vi "Ghost Bus - Tool.vi"() -> ()   [LabVIEW 2019, in "Ghost Bus Tool.lvlib"]
uses:
  Ghost Bus Tool.lvlib
  NationalInstruments.VeriStand.SystemStorage
  SubModules/CAN-Streaming-Support/Source/Addon/Addon Shared/Types/Direction Filter.ctl
  SubModules/CAN-Streaming-Support/Source/Addon/Addon Shared/Types/Type Filter.ctl
  Workspace Shared/Types/Workspace.State.ctl
  Workspace Shared/Types/UI.Refs.ctl
  <vilib>/NI VeriStand/Display Template Support/DisplayTemplateSupport.llb/enum_Display Template Handler Minimal To Workspace.ctl
  Workspace Shared/Types/Workspace.SavedState.ctl
  <vilib>/NI VeriStand/Execution/Workspace/WorkspaceAPI.ctl
  <vilib>/NI VeriStand/Display Template Support/DisplayTemplateSupport.llb/enum_Display Template Handler Minimal To Widget Msg.ctl
  <vilib>/NI VeriStand/Execution/Workspace/SystemStateRegEventRef.ctl
  <vilib>/NI VeriStand/Execution/Workspace/Target State Info.ctl
  <vilib>/NI VeriStand/Execution/Workspace/Target State.ctl
  <vilib>/NI VeriStand/Execution/Workspace/SystemStateEventRef.ctl
  SubModules/CAN-Streaming-Support/Source/UIs/Workspace Shared/Types/Host Stream Queue Refs.ctl
  SubModules/CAN-Streaming-Support/Source/UIs/Workspace Shared/Types/Host Stream Queue Type.ctl
  SubModules/CAN-Streaming-Support/Source/UIs/Workspace Shared/Types/Host Stream Queue Command.ctl
  <vilib>/xnet/xnet.llb/XNET Frame CAN.ctl
  <vilib>/xnet/xnet.llb/XNET Frame Type CAN.ctl
  SubModules/CAN-Streaming-Support/Source/UIs/Workspace Shared/Types/Host Stream Engine Parameters.ctl
  SubModules/CAN-Streaming-Support/Source/Addon/Addon Shared/Types/Filter Parameters.ctl
  <vilib>/Utility/miscctls.llb/LVRowAndColumnUnsignedTypeDef.ctl
  <vilib>/dlg_ctls.llb/Space Constant.vi
  SubModules/CAN-Streaming-Support/Source/UIs/Workspace Shared/SubVIs/Create Host Stream Refs.vi
  SubModules/CAN-Streaming-Support/Source/UIs/Workspace Shared/SubVIs/Read Host Stream.vi
  SubModules/CAN-Streaming-Support/Source/UIs/Workspace Shared/SubVIs/Cleanup Host Stream.vi
  SubModules/CAN-Streaming-Support/Source/UIs/Workspace Shared/SubVIs/Create Bus Log File.vi
  SubModules/CAN-Streaming-Support/Source/UIs/Workspace Shared/SubVIs/Write to Bus Log File.vi
  SubModules/CAN-Streaming-Support/Source/UIs/Workspace Shared/SubVIs/Convert BIN to TXT File.vi
  SubModules/CAN-Streaming-Support/Source/UIs/Workspace Shared/SubVIs/Get Next Bus Engine State.vi
  SubModules/CAN-Streaming-Support/Source/UIs/Workspace Shared/SubVIs/Get Engine Trigger State.vi
  SubModules/CAN-Streaming-Support/Source/UIs/Workspace Shared/SubVIs/Get Next Log Engine State.vi
  SubModules/CAN-Streaming-Support/Source/UIs/Workspace Shared/SubVIs/Process CAN Data.vi
  SubModules/CAN-Streaming-Support/Source/UIs/Workspace Shared/SubVIs/Process CAN State.vi
  SubModules/CAN-Streaming-Support/Source/UIs/Workspace Shared/SubVIs/Convert Frame Array to String Array.vi
  SubModules/CAN-Streaming-Support/Source/UIs/Workspace Shared/SubVIs/Convert Time to UTC String.vi
  <vilib>/Utility/error.llb/Trim Whitespace.vi
  <userlib>/_OpenG.lib/array/array.llb/Sort Array__ogtk.vi
  <userlib>/_OpenG.lib/array/array.llb/Sort 2D Array (String)__ogtk.vi
  <vilib>/Utility/libraryn.llb/Check if File or Folder Exists.vi
  <vilib>/Utility/libraryn.llb/Get File Extension.vi
  Workspace Shared/Ghost Bus Workspace Shared.lvlib
  APIs/Host Automation API/Ghost Bus Host Automation API.lvlib
  <vilib>/NI VeriStand/Execution/Workspace/NI_VS Workspace ExecutionAPI.lvlib
  SubModules/CAN-Streaming-Support/Source/UIs/Workspace Shared/CAN Stream Support Workspace Shared.lvlib
  SubModules/CAN-Streaming-Support/Source/Addon/Addon Shared/CAN Stream Support Shared.lvlib
  NationalInstruments.VeriStand.ClientAPI
panel:
  out "Device":string
  in  "Tab Control":enum32{"Bus Stream", "RAW"}(tab)
  in  "Reset Filter":bool
  in  "Host Filter":bool
  in  "Filter IDs":string caption="Filter IDs (format = x<ID>, comma separated, ID x0 = Bus Error)"
  in  "Clear History":bool
  in  "Type Filter":T1
  out "Table Control":string[][](table)
  in  "Enable Stream":bool
  in  "Pause":bool
  in  "Sort By ID":bool
  out "Stream Connected":bool
  out "Status":string
  in  "Direction Filter":T2
  in  "Log":bool
  in  "Extended?":bool
  in  "Identifier":u32 format="%x"
  in  "Raw Bytes":u8[](array[numeric]) format="%.0x"
  in  "Type":T3(ring)
  out "Error":errorcluster
  in  "Clear Raw":bool
  in  "Send Raw":bool
  in  "NIVS.Gateway IP Address":string
  in  "NIVS.System Definition Root":refnum<k24>
  in  "NIVS.Workspace Event":refnum<event-registration>
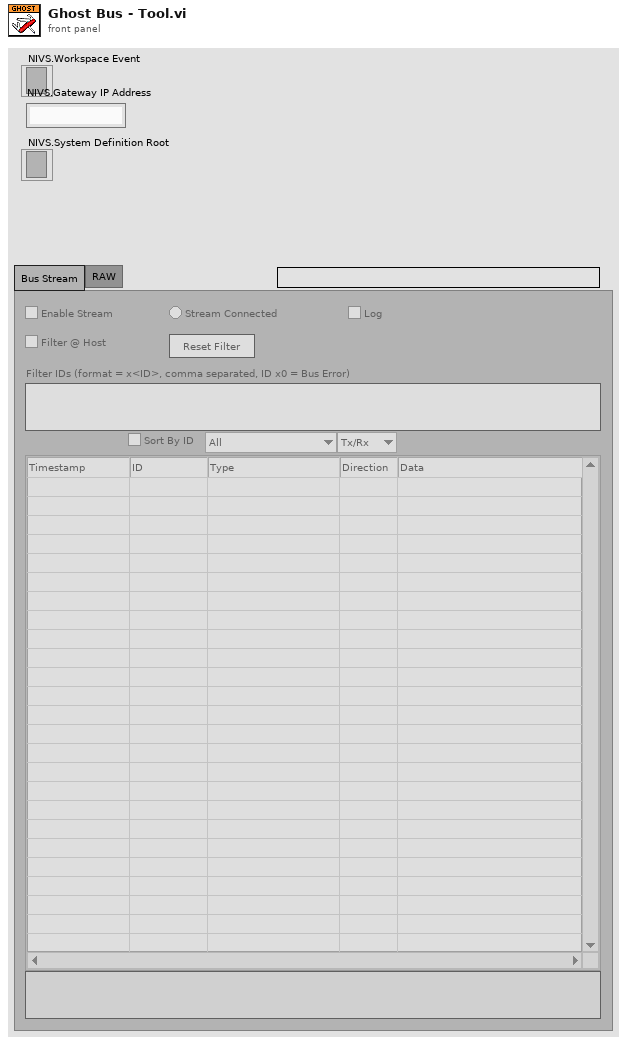
[diagram p1: front panel]
types:
  T1 = typedef "CAN Stream Support Shared.lvlib/Type Filter.ctl" = enum16{"All", "CAN Data", "CAN Remote", "CAN Bus Error", "CAN 2.0 Data", "CAN FD Data", "CAN FD+BRS Data", "J1939 Data", "Delay", "Log Trigger", "Start Trigger"}
  T2 = typedef "CAN Stream Support Shared.lvlib/Direction Filter.ctl" = enum16{"Tx/Rx", "Rx", "Tx"}
  T3 = enum16{"CAN Data", "CAN Remote", "CAN Bus Error", "CAN 2.0 Data", "CAN FD Data", "CAN FD+BRS Data", "J1939 Data", "Delay", "Log Trigger", "Start Trigger"}
  T4 = typedef "Ghost Bus Workspace Shared.lvlib/Workspace.State.ctl" = cluster{"UI.Refs":T5, "CachedData.UserEvent":refnum<user-event>, "CachedData":T6, "Addon.Connected?":bool, "NIVS.SysDef":path, "NIVS.SysDefRoot":refnum<k24>, "NIVS.Workspace":T7, "NIVS.UserEventRefs":cluster{"Event Registration Refnum":refnum<event-registration>, "SystemChangeEventRef":T8, "NIVS.Workspace Event":refnum<event-registration>}, "NIVS.SystemStateRefs":T9, "NIVS.LaunchRef":refnum<user-event>, "Mode.Tool?":bool, "Stream.Qs":T10}
  T5 = typedef "Ghost Bus Workspace Shared.lvlib/UI.Refs.ctl" = cluster{"Device":refnum<vi>, "Pause":refnum<vi>, "Table Control":refnum<vi>, "Sort By ID":refnum<vi>, "Streaming Connected":refnum<vi>, "Enable Stream":refnum<vi>, "CAN State":refnum<vi>, "Direction Filter":refnum<vi>, "Type Filter":refnum<vi>, "Clear History":refnum<vi>, "Filter IDs":refnum<vi>, "Filter Location":refnum<vi>, "Reset Filter":refnum<vi>, "Log":refnum<vi>, "Type":refnum<vi>, "Extended?":refnum<vi>, "Identifier":refnum<vi>, "Raw Bytes":refnum<vi>, "Send Raw":refnum<vi>, "Clear Raw":refnum<vi>, "Raw Error":refnum<vi>}
  T6 = typedef "Ghost Bus Workspace Shared.lvlib/Workspace.SavedState.ctl" = cluster{"CD Path":string, "CD IP":string}
  T7 = typedef "NI_VS Workspace ExecutionAPI.lvlib/WorkspaceAPI.ctl" = refnum<k24>
  T8 = typedef "NI_VS Workspace ExecutionAPI.lvlib/SystemStateRegEventRef.ctl" = refnum<event-registration>
  T9 = typedef "NI_VS Workspace ExecutionAPI.lvlib/SystemStateEventRef.ctl" = cluster{"CustDatRef":refnum<user-event>, "EvtRef":refnum<k27>, "Target State User Event":refnum<user-event>}
  T10 = typedef "CAN Stream Support Workspace Shared.lvlib/Host Stream Queue Refs.ctl" = cluster{"Cmd Q":refnum<queue>, "XNET Frames":refnum<queue>}
  T11 = typedef "enum_Display Template Handler Minimal To Workspace.ctl" = cluster{"Operation":enum16{"SetCustomData", "DeleteItem"}, "Data":variant}
  T12 = typedef "XNET Frame CAN.ctl" = cluster{"timestamp":timestamp, "payload":u8[], "identifier":u32, "type":T13, "extended?":bool, "echo?":bool}
  T13 = typedef "XNET Frame Type CAN.ctl" = u8
  T14 = typedef "CAN Stream Support Shared.lvlib/Filter Parameters.ctl" = cluster{"ID Filters":u32[], "Direction Filter":T2, "Type Filter":T1}
  T15 = typedef "LVRowAndColumnUnsignedTypeDef.ctl" = cluster{"Row":u32, "Column":u32}
  T16 = cluster{"Event Registration Refnum":refnum<event-registration>, "SystemChangeEventRef":T8, "NIVS.Workspace Event":refnum<event-registration>}
  T17 = typedef "enum_Display Template Handler Minimal To Widget Msg.ctl" = enum16{"Stop", "LaunchConfigDialog"}
  T18 = enum8{"Enabled", "Disabled", "Disabled and Grayed Out"}
  T19 = typedef "Ghost Bus Host Automation API.lvlib/API Variables.ctl" = cluster{"TCP Comm":T20}
  T20 = typedef "NI STM.lvlib/TCP Connection Info.ctl" = cluster{"connection ID":refnum<k5>, "meta data":T21[]}
  T21 = typedef "NI STM.lvlib/MetaDataElement.ctl" = string
  T22 = typedef "CAN Stream Support Workspace Shared.lvlib/Host Stream Engine Parameters.ctl" = cluster{"Host Filter":bool, "Filter Parameters":T14, "Sort By ID":bool, "Pause":bool, "Clear History":bool, "Log":bool}
  T23 = typedef "CAN Stream Support Workspace Shared.lvlib/Host Stream Data.ctl" = cluster{"Connected":bool, "Bus Data Update":bool, "Bus Data":string[][], "Bus Status":string, "Bus Warning":bool, "Log Status":string}
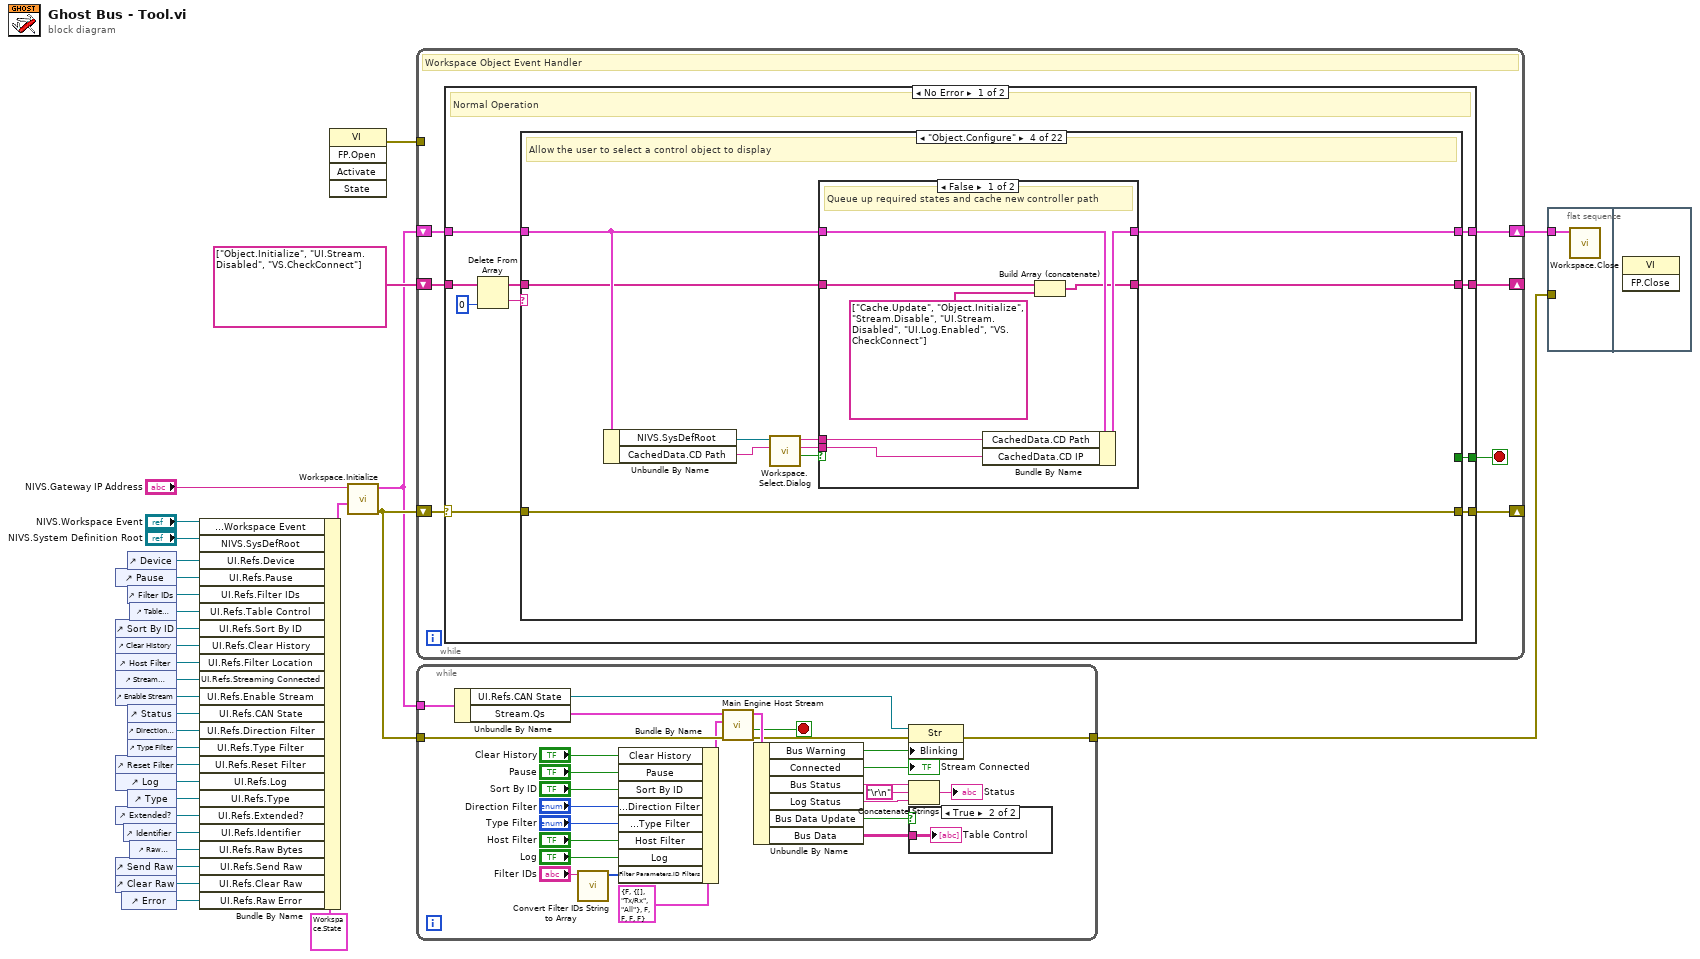
[diagram p0: block diagram]
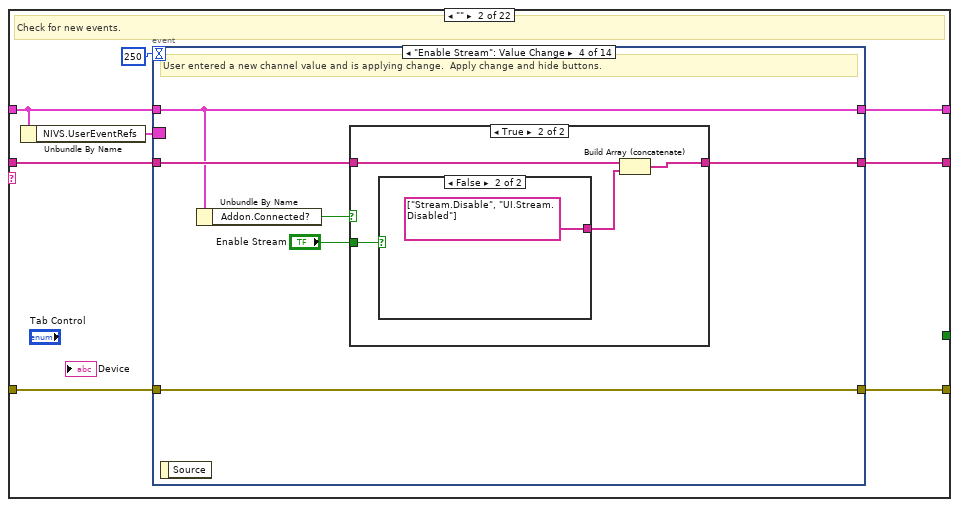
[diagram p4: hidden frame]
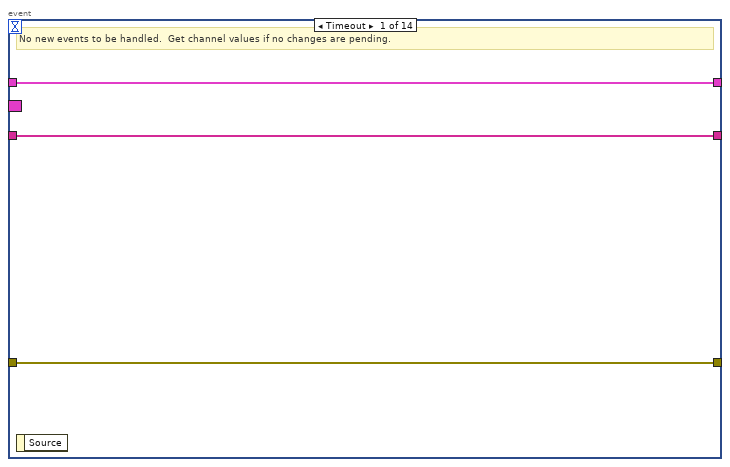
[diagram p5: hidden frame]
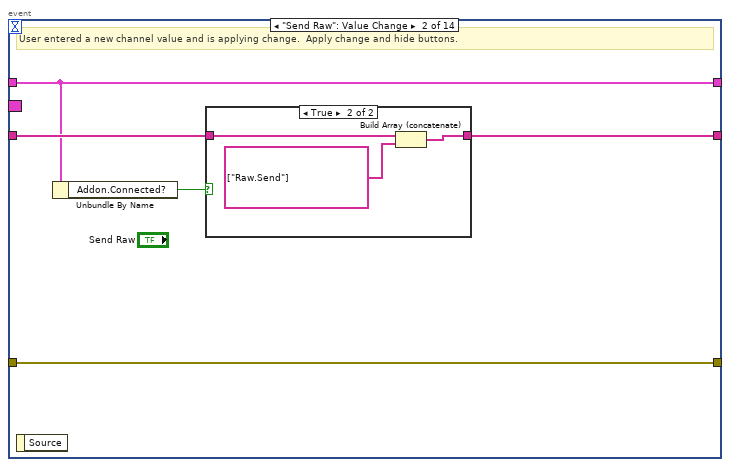
[diagram p6: hidden frame]
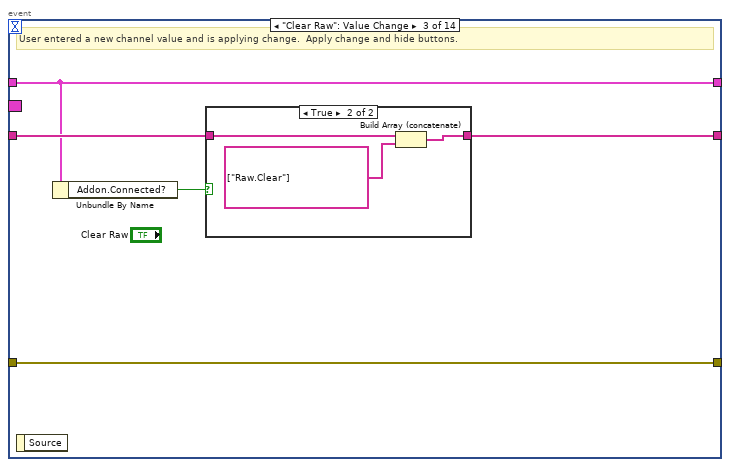
[diagram p8: hidden frame]
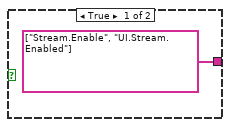
[diagram p11: hidden frame]
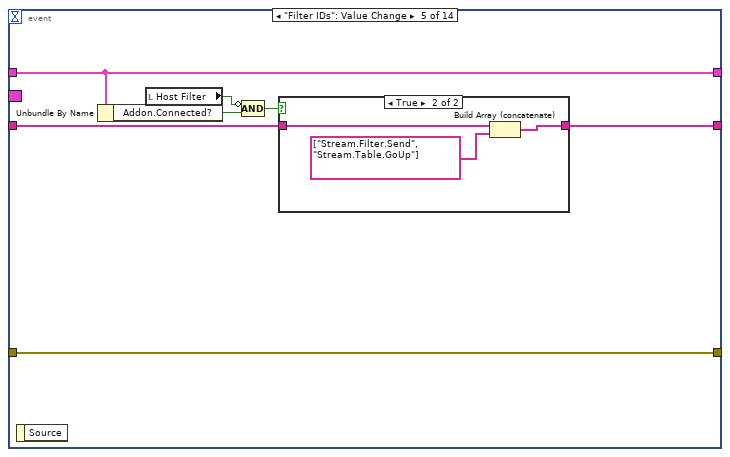
[diagram p12: hidden frame]
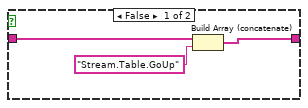
[diagram p13: hidden frame]
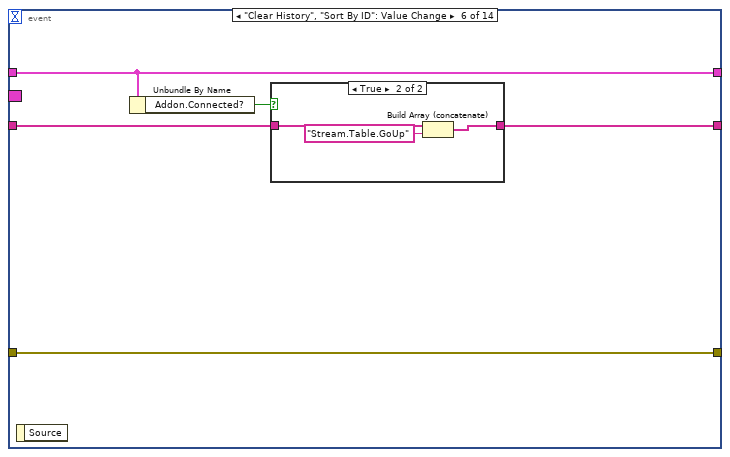
[diagram p14: hidden frame]
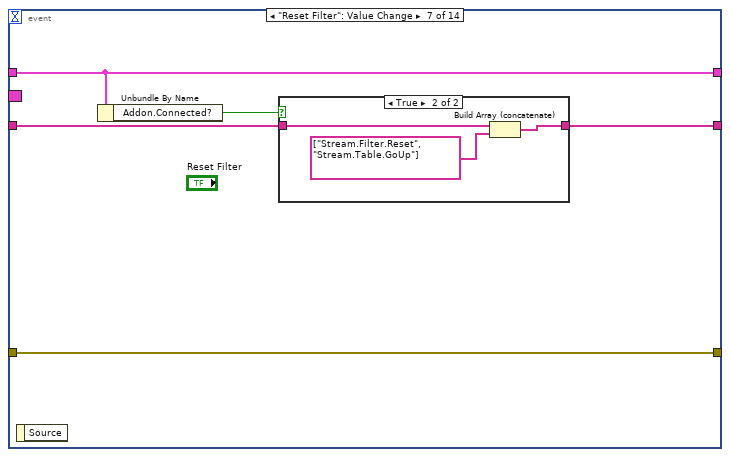
[diagram p16: hidden frame]
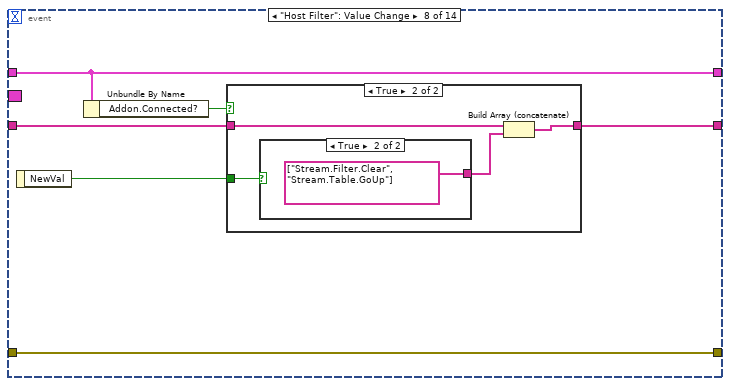
[diagram p18: hidden frame]
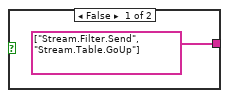
[diagram p20: hidden frame]
diagram:
  n1 = control-ref of="Pause"() -> (w23:refnum<vi>)
  n2 = control-ref of="Sort By ID"() -> (w21:refnum<vi>)
  n3 = control-ref of="Clear History"() -> (w11:refnum<vi>)
  n4 = control-ref of="Host Filter"() -> (w10:refnum<vi>)
  n5 = control-ref of="Stream Connected"() -> (w20:refnum<vi>)
  n6 = control-ref of="Enable Stream"() -> (w19:refnum<vi>)
  n7 = control-ref of="Reset Filter"() -> (w9:refnum<vi>)
  n8 = control-ref of="Log"() -> (w8:refnum<vi>)
  n9 = control-ref of="Extended?"() -> (w4:refnum<vi>)
  n10 = control-ref of="Send Raw"() -> (w1:refnum<vi>)
  n11 = control-ref of="Clear Raw"() -> (w2:refnum<vi>)
  n12 = control-ref of="Error"() -> (w3:refnum<vi>)
  n13 = control-ref of="Identifier"() -> (w5:refnum<vi>)
  n14 = control-ref of="Device"() -> (w24:refnum<vi>)
  n15 = control-ref of="Filter IDs"() -> (w12:refnum<vi>)
  n16 = control-ref of="Status"() -> (w18:refnum<vi>)
  n17 = control-ref of="Direction Filter"() -> (w14:refnum<vi>)
  n18 = control-ref of="Type Filter"() -> (w13:refnum<vi>)
  n19 = control-ref of="Type"() -> (w7:refnum<vi>)
  n20 = control-ref of="Table Control"() -> (w22:refnum<vi>)
  n21 = control-ref of="Raw Bytes"() -> (w6:refnum<vi>)
  n22 = Bundle By Name(cluster=T4 {"UI.Refs"={"Device"=refnum, "Pause"=refnum, "Table Control"=refnum, "Sort By ID"=refnum, "Streaming Connected"=refnum, "Enable Stream"=refnum, "CAN State"=refnum, "Direction Filter"=refnum, "Type Filter"=refnum, "Clear History"=refnum, "Filter IDs"=refnum, "Filter Location"=refnum, "Reset Filter"=refnum, "Log"=refnum, "Type"=refnum, "Extended?"=refnum, "Identifier"=refnum, "Raw Bytes"=refnum, "Send Raw"=refnum, "Clear Raw"=refnum, "Raw Error"=refnum}, "CachedData.UserEvent"=refnum, "CachedData"={"CD Path"="", "CD IP"=""}, "Addon.Connected?"=FALSE, "NIVS.SysDef"=path "", "NIVS.SysDefRoot"=refnum, "NIVS.Workspace"=refnum, "NIVS.UserEventRefs"={"Event Registration Refnum"=refnum, "SystemChangeEventRef"=refnum, "NIVS.Workspace Event"=refnum}, "NIVS.SystemStateRefs"={"CustDatRef"=refnum, "EvtRef"=refnum, "Target State User Event"=refnum}, "NIVS.LaunchRef"=refnum, "Mode.Tool?"=FALSE, "Stream.Qs"={"Cmd Q"=refnum, "XNET Frames"=refnum}}, "NIVS.UserEventRefs.NIVS.Workspace Event"="NIVS.Workspace Event", "NIVS.SysDefRoot"="NIVS.System Definition Root", "UI.Refs.Device"=w24, "UI.Refs.Pause"=w23, "UI.Refs.Filter IDs"=w12, "UI.Refs.Table Control"=w22, "UI.Refs.Sort By ID"=w21, "UI.Refs.Clear History"=w11, "UI.Refs.Filter Location"=w10, "UI.Refs.Streaming Connected"=w20, "UI.Refs.Enable Stream"=w19, "UI.Refs.CAN State"=w18, "UI.Refs.Direction Filter"=w14, "UI.Refs.Type Filter"=w13, "UI.Refs.Reset Filter"=w9, "UI.Refs.Log"=w8, "UI.Refs.Type"=w7, "UI.Refs.Extended?"=w4, "UI.Refs.Identifier"=w5, "UI.Refs.Raw Bytes"=w6, "UI.Refs.Send Raw"=w1, "UI.Refs.Clear Raw"=w2, "UI.Refs.Raw Error"=w3) -> (w30:T4)
  n23 = invoke class="VI" method="FP.Open"() -> (error out=w28:errorcluster)  [unwired: 5 in, 4 out]
  n24 = call "Workspace.Initialize.vi"("State Variables in"=w30, "NIVS.Gateway IP Address"="NIVS.Gateway IP Address") -> ("error out"=w17:errorcluster, "State Variables out"=w16:T4)  [unwired: 8 in]
  n25 = while {
    shift-right: [w37] -> _
    shift-left: string[] ["Object.Initialize", "UI.Stream.Disabled", "VS.CheckConnect"] -> [w38]
    shift-right: [w35] -> w27
    shift-left: w16 -> [w34]
    shift-right: [w36] -> _
    shift-left: w17 -> [w33]
    tunnel: w28 -> [_]
    stop <- w39 stop-if-true
    # "Workspace Object Event Handler"
    n26 = case shown="No Error" w33 {
      selector: w33 -> [w40 w431]
      tunnel: [w49 _] -> w39
      tunnel: w38 -> [w47 w438]
      tunnel: [w44 w438] -> w37
      tunnel: [w43 w429] -> w36
      tunnel: [w42 w437] -> w35
      tunnel: w34 -> [w41 w437]
      frame No Error {
        # "Normal Operation"
        n27 = Delete From Array(array=w47, index=0) -> (deleted portion=w46:string, array with subset deleted=w45:string[])  [unwired: 1 in]
        n28 = case shown="\"Object.Configure\"" w46 {
          tunnel: [_ _ _ _ _ _ _ TRUE _ _ _ _ _ _ _ _ _ _ _ _ _ _] -> w49
          tunnel: [w52 w59 w210 w215 w236 w242 w248 w269 w276 w280 w294 w307 w320 w341 w345 w354 w372 w384 w401 w417 w423 w428] -> w44
          tunnel: w40 -> [w51 w57 w205 w221 w231 w240 w253 w266 w275 w278 w291 w305 w317 w340 w344 w353 w365 w377 w394 w408 w418 w424]
          tunnel: w45 -> [w52 w58 w210 w214 w236 w242 w247 w269 w276 w280 w294 w307 w320 w341 w345 w354 w372 w384 w401 w417 w423 w428]
          tunnel: w41 -> [w50 w53 w209 w219 w232 w239 w245 w265 w272 w277 w293 w306 w319 w337 w343 w351 w368 w380 w397 w411 w422 w427]
          tunnel: [w51 w56 w207 w221 w234 w237 w252 w267 w275 w279 w282 w304 w309 w340 w344 w352 w365 w377 w394 w408 w419 w425] -> w43
          tunnel: [w50 w55 w209 w218 w233 w238 w246 w265 w272 w277 w293 w306 w319 w337 w343 w351 w368 w380 w397 w411 w422 w427] -> w42
          frame Default {
            # "Do nothing."
          }
          frame "" {
            # "Check for new events."
            n29 = Unbundle By Name(w53) -> ("NIVS.UserEventRefs"=w54:T16)
            n30 = event shown="[3] \"Enable Stream\": Value Change" {
              selector: w54 -> [_ _ _ _ _ _ _ _ _ _ _ _ _ _]
              dyn-events: _ -> [_ _ _ _ _ _ _ _ _ _ _ _ _ _]
              timeout: 250 -> [_ _ _ _ _ _ _ _ _ _ _ _ _ _]
              tunnel: [w61 w66 w75 w85 w100 w111 w120 w130 w143 w153 w166 w182 w194 w201] -> w59
              tunnel: w58 -> [w61 w67 w76 w86 w99 w110 w119 w129 w142 w155 w165 w181 w195 w202]
              tunnel: w57 -> [w63 w68 w77 w87 w101 w112 w121 w131 w144 w152 w173 w180 w198 w204]
              tunnel: [w63 w68 w77 w87 w101 w112 w121 w131 w144 w152 w173 w180 w198 w204] -> w56
              tunnel: [w62 w65 w74 w84 w98 w109 w118 w128 w141 w157 w172 w178 w197 w203] -> w55
              tunnel: w53 -> [w62 w65 w74 w84 w98 w109 w118 w128 w141 w157 w172 w179 w197 w203]
              event Timeout {
                # "No new events to be handled.  Get channel values if no changes are pending."
                n31 = event-data() -> ()  [unwired: 2 out]
              }
              event "Send Raw": Value Change {
                # "User entered a new channel value and is applying change.  Apply change and hide buttons."
                n32 = event-data() -> ()  [unwired: 2 out]
                n33 = Unbundle By Name(w65) -> ("Addon.Connected?"=w64:bool)
                n34 = case shown="True" w64 {
                  tunnel: w67 -> [w69 w71]
                  tunnel: [w69 w70] -> w66
                  frame False {
                  }
                  frame True {
                    n35 = Build Array (concatenate)(w71, string[] ["Raw.Send"]) -> (w70:string[])
                  }
                }
              }
              event "Clear Raw": Value Change {
                # "User entered a new channel value and is applying change.  Apply change and hide buttons."
                n36 = event-data() -> ()  [unwired: 2 out]
                n37 = Unbundle By Name(w74) -> ("Addon.Connected?"=w73:bool)
                n38 = case shown="True" w73 {
                  tunnel: w76 -> [w78 w80]
                  tunnel: [w78 w79] -> w75
                  frame False {
                  }
                  frame True {
                    n39 = Build Array (concatenate)(w80, string[] ["Raw.Clear"]) -> (w79:string[])
                  }
                }
              }
              event "Enable Stream": Value Change {
                # "User entered a new channel value and is applying change.  Apply change and hide buttons."
                n40 = event-data() -> ()  [unwired: 2 out]
                n41 = Unbundle By Name(w84) -> ("Addon.Connected?"=w83:bool)
                n42 = case shown="True" w83 {
                  tunnel: w86 -> [w88 w91]
                  tunnel: [w88 w90] -> w85
                  tunnel: "Enable Stream" -> [_ w89]
                  frame False {
                  }
                  frame True {
                    n43 = case shown="False" w89 {
                      tunnel: [string[] ["Stream.Enable", "UI.Stream.Enabled"] string[] ["Stream.Disable", "UI.Stream.Disabled"]] -> w92
                      frame True {
                      }
                      frame False {
                      }
                    }
                    n44 = Build Array (concatenate)(w91, w92) -> (w90:string[])
                  }
                }
              }
              event "Filter IDs": Value Change {
                n45 = event-data() -> ()  [unwired: 2 out]
                n46 = Unbundle By Name(w98) -> ("Addon.Connected?"=w96:bool)
                n47 = local read "Host Filter"() -> (w97:bool)
                n48 = Compound Arithmetic op=AND(invert w97, w96) -> (w95:bool)
                n49 = case shown="True" w95 {
                  tunnel: w99 -> [w102 w106]
                  tunnel: [w103 w105] -> w100
                  frame False {
                    n50 = Build Array (concatenate)(w102, "Stream.Table.GoUp") -> (w103:string[])
                  }
                  frame True {
                    n51 = Build Array (concatenate)(w106, string[] ["Stream.Filter.Send", "Stream.Table.GoUp"]) -> (w105:string[])
                  }
                }
              }
              event "Clear History", "Sort By ID": Value Change {
                n52 = event-data() -> ()  [unwired: 2 out]
                n53 = Unbundle By Name(w109) -> ("Addon.Connected?"=w108:bool)
                n54 = case shown="True" w108 {
                  tunnel: [w113 w116] -> w111
                  tunnel: w110 -> [w113 w115]
                  frame False {
                  }
                  frame True {
                    n55 = Build Array (concatenate)(w115, "Stream.Table.GoUp") -> (w116:string[])
                  }
                }
              }
              event "Reset Filter": Value Change {
                n56 = event-data() -> ()  [unwired: 2 out]
                n57 = Unbundle By Name(w118) -> ("Addon.Connected?"=w117:bool)
                n58 = case shown="True" w117 {
                  tunnel: w119 -> [w122 w124]
                  tunnel: [w122 w123] -> w120
                  frame False {
                  }
                  frame True {
                    n59 = Build Array (concatenate)(w124, string[] ["Stream.Filter.Reset", "Stream.Table.GoUp"]) -> (w123:string[])
                  }
                }
              }
              event "Host Filter": Value Change {
                n60 = event-data() -> ("NewVal"=w126:bool)  [unwired: 1 out]
                n61 = Unbundle By Name(w128) -> ("Addon.Connected?"=w127:bool)
                n62 = case shown="True" w127 {
                  tunnel: w129 -> [w132 w135]
                  tunnel: [w132 w134] -> w130
                  tunnel: w126 -> [_ w133]
                  frame False {
                  }
                  frame True {
                    n63 = case shown="True" w133 {
                      tunnel: [string[] ["Stream.Filter.Send", "Stream.Table.GoUp"] string[] ["Stream.Filter.Clear", "Stream.Table.GoUp"]] -> w136
                      frame False {
                      }
                      frame True {
                      }
                    }
                    n64 = Build Array (concatenate)(w135, w136) -> (w134:string[])
                  }
                }
              }
              event "Log": Value Change {
                n65 = event-data() -> ("NewVal"=w139:bool)  [unwired: 1 out]
                n66 = Unbundle By Name(w141) -> ("Addon.Connected?"=w140:bool)
                n67 = case shown="True" w140 {
                  tunnel: w142 -> [w145 w148]
                  tunnel: [w145 w147] -> w143
                  tunnel: w139 -> [_ w146]
                  frame False {
                  }
                  frame True {
                    n68 = case shown="False" w146 {
                      tunnel: [string[] ["UI.Log.Disabled"] string[] ["UI.Log.Enabled"]] -> w149
                      frame False {
                      }
                      frame True {
                      }
                    }
                    n69 = Build Array (concatenate)(w148, w149) -> (w147:string[])
                  }
                }
              }
              event User Event {
                # "System state has changed. Handle accordingly."
                n70 = event-data() -> ("SystemStateChange"=w156:string)  [unwired: 1 out]
                n71 = Unbundle By Name(w157) -> ("Mode.Tool?"=w158:bool)
                n72 = case shown="True" w158 {
                  tunnel: ["VS.CheckConnect" w161] -> w154
                  tunnel: w156 -> [_ w160]
                  frame False {
                  }
                  frame True {
                    n73 = case shown="\"Stop Configuration\"" w160 {
                      tunnel: ["Object.Exit" "VS.CheckConnect"] -> w161
                      frame "Stop Configuration" {
                      }
                      frame Default {
                      }
                    }
                  }
                }
                n74 = Build Array (concatenate)(w155, w154) -> (w153:string[])
              }
              event User Event {
                n75 = event-data() -> ("Workspace Event"=w167:string)  [unwired: 1 out]
                n76 = Equal?(x=w167, y="Shut Down") -> (x = y?=w168:bool)
                n77 = Equal?(x=w167, y="Disconnect") -> (x = y?=w169:bool)
                n78 = Compound Arithmetic op=OR(w168, w169) -> (w164:bool)
                n79 = case shown="True" w164 {
                  tunnel: [w174 w176] -> w166
                  tunnel: w165 -> [w174 w175]
                  frame False {
                  }
                  frame True {
                    n80 = Build Array (concatenate)(w175, "Object.Exit") -> (w176:string[])
                  }
                }
              }
              event User Event {
                # "Widget event has occurred.  Handle accordingly."
                n81 = event-data() -> ("ToWidgetMessage"=w183:T17)  [unwired: 1 out]
                n82 = case shown="\"Stop\"" w183 {
                  tunnel: [w185 w188 w192] -> w182
                  tunnel: w181 -> [w185 w189 w193]
                  tunnel: w179 -> [w184 w186 w190]
                  tunnel: [w184 w186 w190] -> w178
                  frame Default {
                    # "Do nothing."
                  }
                  frame "Stop" {
                    # "User exiting workspace or deleting object"
                    n83 = Build Array (concatenate)(w189, "Object.Exit") -> (w188:string[])
                  }
                  frame "LaunchConfigDialog" {
                    # "User wants to configure object"
                    n84 = Build Array (concatenate)(w193, "Object.Configure") -> (w192:string[])
                  }
                }
              }
              event Menu Selection (User) {
                n85 = event-data() -> ("ItemTag"=w196:string)  [unwired: 1 out]
                n86 = Build Array (concatenate)(w195, w196) -> (w194:string[])
              }
              event Panel Close? {
                n87 = event-data() -> ()  [unwired: 5 out]
                n88 = Build Array (concatenate)(w202, "Object.Exit") -> (w201:string[])
                n89 = event-data("Discard?"=TRUE) -> ()  [unwired: 1 in, 1 out]
              }
            }
          }
          frame "Object.Initialize" {
            # "Initialize the workspace Object state variables and UI"
            n90 = local write "Tab Control"(0) -> ()
            n91 = Unbundle By Name(w209) -> ("UI.Refs.Filter Location"=w206:refnum<vi>)
            n92 = property class="Bool (strict)"(reference=w206, error in=w205, "Value"=FALSE) -> (error out=w207:errorcluster)  [unwired: 1 out]
          }
          frame "Object.Configure" {
            # "Allow the user to select a control object to display"
            n93 = Unbundle By Name(w219) -> ("NIVS.SysDefRoot"=w213:refnum<k24>, "CachedData.CD Path"=w220:string)
            n94 = call "Workspace.Select.Dialog.vi"("CD Path"=w220, "NIVS.System Definition Root"=w213) -> ("Cancelled?"=w217:bool, "IP Address"=w212:string, "Custom Device Path Out"=w216:string)  [unwired: 7 in]
            n95 = case shown="False" w217 {
              tunnel: w219 -> [w228 w229]
              tunnel: [w227 w229] -> w218
              tunnel: w216 -> [w226 _]
              tunnel: [w224 w230] -> w215
              tunnel: w214 -> [w225 w230]
              tunnel: w212 -> [w222 _]
              frame False {
                # "Queue up required states and cache new controller path"
                n96 = Bundle By Name(cluster=w228, "CachedData.CD Path"=w226, "CachedData.CD IP"=w222) -> (w227:T4)
                n97 = Build Array (concatenate)(w225, string[] ["Cache.Update", "Object.Initialize", "Stream.Disable", "UI.Stream.Disabled", "UI.Log.Enabled", "VS.CheckConnect"]) -> (w224:string[])
              }
              frame True {
                # "User canceled"
              }
            }
          }
          frame "Object.Connected" {
            # "System state is Connected. Get path to required channels and start UDP acquisition if channels found."
            n98 = call "Workspace.UI.DisableState.Set.vi"("Enable?"=TRUE, "error in (no error)"=w231, "State Variables in"=w232) -> ("error out"=w234:errorcluster, "State Variables out"=w233:T4)  [unwired: 7 in]
          }
          frame "Object.Disconnected" {
            n99 = call "Workspace.UI.DisableState.Set.vi"("Enable?"=FALSE, "error in (no error)"=w240, "State Variables in"=w239) -> ("error out"=w237:errorcluster, "State Variables out"=w238:T4)  [unwired: 7 in]
          }
          frame "VS.CheckConnect" {
            n100 = Unbundle By Name(w245) -> ("UI.Refs.Device"=w244:refnum<vi>, "NIVS.Workspace"=w256:T7, "NIVS.SysDefRoot"=w255:refnum<k24>, "CachedData.CD Path"=w254:string)
            n101 = Current VI's Menubar() -> (w257:refnum<k9>)
            n102 = call "UI.Connection.State.Get.vi"("Menu Ref"=w257, "Name Ref"=w244, "error in (no error)"=w253, "Addon Path in"=w254, "NIVS.System Definition Root in"=w255, "NIVS.Workspace Ref in"=w256) -> ("error out"=w252:errorcluster, "Addon Connected?"=w249:bool, "NIVS.System Definition Root out"=w250:refnum<k24>, "NIVS.Workspace Ref out"=w251:T7, "System Definition File"=w243:path)  [unwired: 1 in]
            n103 = case shown="True" w249 {
              tunnel: [w260 w263] -> w248
              tunnel: w247 -> [w259 w262]
              frame True {
                # "Addon connected"
                n104 = Build Array (concatenate)(w259, string[] ["Object.Connected", "Stream.Filter.Read"]) -> (w260:string[])
              }
              frame False {
                # "Addon not connected"
                n105 = Build Array (concatenate)(w262, string[] ["Object.Disconnected", "UI.Stream.Disabled", "Stream.Disable"]) -> (w263:string[])
              }
            }
            n106 = Bundle By Name(cluster=w245, "NIVS.SysDef"=w243, "NIVS.Workspace"=w251, "NIVS.SysDefRoot"=w250, "Addon.Connected?"=w249) -> (w246:T4)
          }
          frame "Object.Exit" {
            # "Stop current loop.  Queue Stop Acq and Exit to UDP loop."
            n107 = Unbundle By Name(w265) -> ("Stream.Qs"=w264:T10)
            n108 = call "Send Host Stream Command Exit.vi"("error in (no error)"=w266, "Q Refs"=w264) -> ("error out"=w267:errorcluster)  [unwired: 9 in]
          }
          frame "Cache.Update" {
            # "Cache any data needing to be permenantly stored with the workspace object."
            n109 = Unbundle By Name(w272) -> ("CachedData.UserEvent"=w270:refnum<user-event>, "CachedData"=w271:T6)
            n110 = Bundle By Name(cluster=T11 {"Operation"=enum."SetCustomData", "Data"=variant} ("event data"), "Data"=w271) -> (w273:T11)
            n111 = Generate User Event(user event=w270, event data cluster=w273) -> ()  [unwired: 2 in, 2 out]
          }
          frame "UI.Stream.Enabled" {
            n112 = call "UI.Stream.Enable.vi"("error in (no error)"=w278, "State Variables in"=w277) -> ("error out"=w279:errorcluster)  [unwired: 9 in]
          }
          frame "UI.Log.Enabled" {
            w281 = T18."Disabled and Grayed Out" ("Disabled")
            n113 = Unbundle By Name(w293) -> ("UI.Refs.Type Filter"=w286:refnum<vi>, "UI.Refs.Filter IDs"=w285:refnum<vi>, "UI.Refs.Direction Filter"=w284:refnum<vi>, "UI.Refs.Reset Filter"=w289:refnum<vi>, "UI.Refs.Filter Location"=w292:refnum<vi>)
            n114 = property class="Bool (strict)"(reference=w292, error in=w291, "DisabledEnum"=w281) -> (error out=w290:errorcluster, "Value"=w288:bool)  [unwired: 1 out]
            n115 = Build Array(w286, w285, w284) -> (w283:refnum<vi>[])
            n116 = property class="Bool"(reference=w289, error in=w290, "DisabledEnum"=w281) -> (error out=w287:errorcluster)  [unwired: 1 out]
            n117 = case shown="False" w288 {
              tunnel: w287 -> [w297 w303]
              tunnel: w283 -> [w298 _]
              tunnel: [w296 w303] -> w282
              tunnel: w281 -> [w295 _]
              frame False {
                n118 = for {
                  tunnel: w298 -> [w302] mode=indexing
                  shift-right: [w300] -> w296
                  shift-left: w297 -> [w301]
                  tunnel: w295 -> [w299]
                  n119 = property class="Ctl"(reference=w302, error in=w301, "DisabledEnum"=w299) -> (error out=w300:errorcluster)  [unwired: 1 out]
                }
              }
              frame True {
              }
            }
          }
          frame "UI.Stream.Disabled" {
            n120 = call "UI.Stream.Disable.vi"("error in (no error)"=w305, "State Variables in"=w306) -> ("error out"=w304:errorcluster)  [unwired: 9 in]
          }
          frame "UI.Log.Disabled" {
            w308 = T18."Enabled" ("Disabled")
            n121 = Unbundle By Name(w319) -> ("UI.Refs.Type Filter"=w313:refnum<vi>, "UI.Refs.Filter IDs"=w312:refnum<vi>, "UI.Refs.Direction Filter"=w311:refnum<vi>, "UI.Refs.Reset Filter"=w315:refnum<vi>, "UI.Refs.Filter Location"=w318:refnum<vi>)
            n122 = property class="Bool (strict)"(reference=w318, error in=w317, "DisabledEnum"=w308) -> (error out=w316:errorcluster)  [unwired: 1 out]
            n123 = Build Array(w313, w312, w311) -> (w310:refnum<vi>[])
            n124 = property class="Bool"(reference=w315, error in=w316, "DisabledEnum"=w308) -> (error out=w314:errorcluster)  [unwired: 1 out]
            n125 = for {
              tunnel: w310 -> [w324] mode=indexing
              shift-right: [w322] -> w309
              shift-left: w314 -> [w323]
              tunnel: w308 -> [w321]
              n126 = property class="Ctl"(reference=w324, error in=w323, "DisabledEnum"=w321) -> (error out=w322:errorcluster)  [unwired: 1 out]
            }
          }
          frame "Raw.Send" {
            # "Reset slow speed channel displayed values."
            n127 = Unbundle By Name(w337) -> ("CachedData.CD IP"=w335:string, "CachedData.CD Path"=w333:string)
            n128 = call "UI.Addon.Path.Parse.vi"("Cached Addon Path"=w333) -> ("Addon Name"=w332:string)  [unwired: 6 in, 4 out]
            n129 = call "Connect.vi"("Addon Name"=w332, "Address"=w335) -> ("error out"=w336:errorcluster, "Ref"=w338:T19)  [unwired: 8 in]
            n130 = Bundle By Name(cluster=T12 {"timestamp"=timestamp(0 s since 1904-01-01), "payload"=[], "identifier"=0, "type"=0, "extended?"=FALSE, "echo?"=FALSE} ("Frame"), "extended?"="Extended?", "type"="Type", "identifier"="Identifier", "payload"="Raw Bytes") -> (w330:T12)
            n131 = call "PassThru.vi"("error in (no error)"=w336, "timeout ms (1000)"=2500, "Frame"=w330, "Ref in"=w338) -> ("error out"=w331:errorcluster, "Ref out"=w339:T19)  [unwired: 6 in]
            "Error" <- w331
            n132 = call "Disconnect.vi"("error in (no error)"=w331, "Ref"=w339) -> ()  [unwired: 9 in, 1 out]
          }
          frame "Raw.Clear" {
            n133 = local write "Raw Bytes"(u8[] [] ("Cmd")) -> ()
          }
          frame "Stream.Enable" {
            n134 = Unbundle By Name(w351) -> ("Stream.Qs"=w348:T10, "CachedData.CD IP"=w349:string, "CachedData.CD Path"=w355:string, "NIVS.SysDef"=w347:path)
            n135 = Strip Path(path=w347) -> (stripped path=w346:path)  [unwired: 1 out]
            n136 = call "UI.Addon.Path.Parse.vi"("Cached Addon Path"=w355) -> ("Addon Name"=w350:string)  [unwired: 6 in, 4 out]
            n137 = call "Send Host Stream Command Start.vi"("Project Folder"=w346, "error in (no error)"=w353, "Addon"=w350, "Target IP Address"=w349, "Q Refs"=w348) -> ("error out"=w352:errorcluster)  [unwired: 6 in]
          }
          frame "Stream.Filter.Send" {
            n138 = Unbundle By Name(w368) -> ("CachedData.CD IP"=w366:string, "CachedData.CD Path"=w369:string)
            n139 = local read "Direction Filter"() -> (w357:T2)
            n140 = local read "Type Filter"() -> (w358:T1)
            n141 = local read "Filter IDs"() -> (w359:string)
            n142 = call "Convert Filter IDs String to Array.vi"("Filter IDs"=w359) -> ("Filter IDs"=w356:u32[])  [unwired: 10 in]
            n143 = call "UI.Addon.Path.Parse.vi"("Cached Addon Path"=w369) -> ("Addon Name"=w367:string)  [unwired: 6 in, 4 out]
            n144 = Bundle By Name(cluster=T14 {"ID Filters"=[], "Direction Filter"=enum."Tx/Rx", "Type Filter"=enum."All"} ("IDs"), "Direction Filter"=w357, "Type Filter"=w358, "ID Filters"=w356) -> (w360:T14)
            n145 = call "Connect.vi"("Addon Name"=w367, "Address"=w366) -> ("error out"=w363:errorcluster, "Ref"=w362:T19)  [unwired: 8 in]
            n146 = call "SetStreamingFilter.vi"("error in (no error)"=w363, "IDs"=w360, "Ref in"=w362) -> ("error out"=w371:errorcluster, "Ref out"=w370:T19)  [unwired: 7 in]
            n147 = call "Disconnect.vi"("error in (no error)"=w371, "Ref"=w370) -> ("error out"=w364:errorcluster)  [unwired: 9 in]
            n148 = call <vilib>:"Simple Error Handler.vi"("error in (no error)"=w364) -> ()  [unwired: 4 in, 5 out]
          }
          frame "Stream.Filter.Clear" {
            n149 = Unbundle By Name(w380) -> ("CachedData.CD IP"=w378:string, "CachedData.CD Path"=w381:string)
            n150 = call "UI.Addon.Path.Parse.vi"("Cached Addon Path"=w381) -> ("Addon Name"=w379:string)  [unwired: 6 in, 4 out]
            n151 = call "Connect.vi"("Addon Name"=w379, "Address"=w378) -> ("error out"=w375:errorcluster, "Ref"=w374:T19)  [unwired: 8 in]
            n152 = call "SetStreamingFilter.vi"("error in (no error)"=w375, "IDs"=T14 {"ID Filters"=[], "Direction Filter"=enum."Tx/Rx", "Type Filter"=enum."All"}, "Ref in"=w374) -> ("error out"=w383:errorcluster, "Ref out"=w382:T19)  [unwired: 7 in]
            n153 = call "Disconnect.vi"("error in (no error)"=w383, "Ref"=w382) -> ("error out"=w376:errorcluster)  [unwired: 9 in]
            n154 = call <vilib>:"Simple Error Handler.vi"("error in (no error)"=w376) -> ()  [unwired: 4 in, 5 out]
          }
          frame "Stream.Filter.Reset" {
            n155 = Unbundle By Name(w397) -> ("CachedData.CD IP"=w395:string, "CachedData.CD Path"=w398:string)
            n156 = call "UI.Addon.Path.Parse.vi"("Cached Addon Path"=w398) -> ("Addon Name"=w396:string)  [unwired: 6 in, 4 out]
            n157 = call "Connect.vi"("Addon Name"=w396, "Address"=w395) -> ("error out"=w392:errorcluster, "Ref"=w391:T19)  [unwired: 8 in]
            n158 = call "ResetStreamingFilter.vi"("error in (no error)"=w392, "Ref in"=w391) -> ("error out"=w400:errorcluster, "IDs"=w387:T14, "Ref out"=w399:T19)  [unwired: 7 in]
            n159 = local write "Host Filter"(FALSE ("Host Filter")) -> ()
            n160 = Unbundle By Name(w387) -> ("ID Filters"=w386:u32[], "Direction Filter"=w389:T2, "Type Filter"=w388:T1)
            n161 = call "Disconnect.vi"("error in (no error)"=w400, "Ref"=w399) -> ("error out"=w393:errorcluster)  [unwired: 9 in]
            n162 = call <vilib>:"Simple Error Handler.vi"("error in (no error)"=w393) -> ()  [unwired: 4 in, 5 out]
            n163 = call "Convert Filter IDs Array to String.vi"("Filter IDs"=w386) -> ("Filter IDs"=w385:string)  [unwired: 10 in]
            n164 = local write "Filter IDs"(w385) -> ()
            n165 = local write "Direction Filter"(w389) -> ()
            n166 = local write "Type Filter"(w388) -> ()
          }
          frame "Stream.Filter.Read" {
            n167 = Unbundle By Name(w411) -> ("CachedData.CD IP"=w409:string, "CachedData.CD Path"=w412:string)
            n168 = call "UI.Addon.Path.Parse.vi"("Cached Addon Path"=w412) -> ("Addon Name"=w410:string)  [unwired: 6 in, 4 out]
            n169 = call "Connect.vi"("Addon Name"=w410, "Address"=w409) -> ("error out"=w415:errorcluster, "Ref"=w416:T19)  [unwired: 8 in]
            n170 = call "GetStreamingFilter.vi"("error in (no error)"=w415, "Ref in"=w416) -> ("error out"=w414:errorcluster, "IDs"=w406:T14, "Ref out"=w413:T19)  [unwired: 7 in]
            n171 = Unbundle By Name(w406) -> ("ID Filters"=w403:u32[], "Direction Filter"=w405:T2, "Type Filter"=w404:T1)
            n172 = call "Disconnect.vi"("error in (no error)"=w414, "Ref"=w413) -> ("error out"=w407:errorcluster)  [unwired: 9 in]
            n173 = call <vilib>:"Simple Error Handler.vi"("error in (no error)"=w407) -> ()  [unwired: 4 in, 5 out]
            n174 = local write "Direction Filter"(w405) -> ()
            n175 = local write "Type Filter"(w404) -> ()
            n176 = call "Convert Filter IDs Array to String.vi"("Filter IDs"=w403) -> ("Filter IDs"=w402:string)  [unwired: 10 in]
            n177 = local write "Filter IDs"(w402) -> ()
          }
          frame "Stream.Table.GoUp" {
            n178 = Unbundle By Name(w422) -> ("UI.Refs.Table Control"=w420:refnum<vi>)
            n179 = property class="Tbl (strict)"(reference=w420, error in=w418, "Index Values"=T15 {"Row"=0, "Column"=0}) -> (error out=w419:errorcluster)  [unwired: 1 out]
          }
          frame "Stream.Disable" {
            n180 = Unbundle By Name(w427) -> ("Stream.Qs"=w426:T10)
            n181 = call "Send Host Stream Command Stop.vi"("error in (no error)"=w424, "Q Refs"=w426) -> ("error out"=w425:errorcluster)  [unwired: 9 in]
          }
        }
      }
      frame Error {
        # "Handle Errors."
        n182 = Unbundle By Name(w431) -> ("code"=w435:i32)
        n183 = Equal?(x=-307654, y=w435) -> (x = y?=w433:bool)
        n184 = Select(t=errorcluster {"status"=FALSE, "code"=0, "source"=""}, s=w433, f=w431) -> (s? t:f=w430:errorcluster)
        n185 = call <vilib>:"Simple Error Handler.vi"("error in (no error)"=w430) -> ("error out"=w436:errorcluster)  [unwired: 4 in, 4 out]
        n186 = call <vilib>:"Clear Errors.vi"("error in (no error)"=w436) -> ("error out"=w429:errorcluster)  [unwired: 5 in, 1 out]
      }
    }
  }
  n187 = while {
    tunnel: w17 -> [w465]
    tunnel: w16 -> [w464]
    tunnel: [w458] -> w15
    stop <- w457 stop-if-true
    n188 = Unbundle By Name(w464) -> ("UI.Refs.CAN State"=w462:refnum<vi>, "Stream.Qs"=w463:T10)
    n189 = call "Convert Filter IDs String to Array.vi"("Filter IDs"="Filter IDs") -> ("Filter IDs"=w440:u32[])  [unwired: 10 in]
    n190 = Bundle By Name(cluster=T22 {"Host Filter"=FALSE, "Filter Parameters"={"ID Filters"=[], "Direction Filter"=enum."Tx/Rx", "Type Filter"=enum."All"}, "Sort By ID"=FALSE, "Pause"=FALSE, "Clear History"=FALSE, "Log"=FALSE} ("Host Parameters"), "Clear History"="Clear History", "Pause"="Pause", "Sort By ID"="Sort By ID", "Filter Parameters.Direction Filter"="Direction Filter", "Filter Parameters.Type Filter"="Type Filter", "Host Filter"="Host Filter", "Log"="Log", "Filter Parameters.ID Filters"=w440) -> (w452:T22)
    n191 = call "Main Engine Host Stream.vi"("error in (no error)"=w465, "Host Parameters"=w452, "Q Refs"=w463) -> ("error out"=w439:errorcluster, "Exit"=w457:bool, "Stream"=w461:T23)  [unwired: 6 in]
    n192 = Unbundle By Name(w461) -> ("Bus Warning"=w460:bool, "Connected"=→"Stream Connected":bool, "Bus Status"=w451:string, "Log Status"=w447:string, "Bus Data Update"=w446:bool, "Bus Data"=w445:string[][])
    n193 = property class="Str"(reference=w462, error in=w439, "Blinking"=w460) -> (error out=w458:errorcluster)  [unwired: 1 out]
    n194 = Concatenate Strings(w451, "\r\n", w447) -> (→"Status":string)
    n195 = case shown="True" w446 {
      tunnel: w445 -> [_ w466]
      frame False {
      }
      frame True {
        "Table Control" <- w466
      }
    }
  }
  n196 = flat-sequence {
    tunnel: w27 -> [w467]
    tunnel: w15 -> [_]
    frame #0 {
      n197 = call "Workspace.Close.vi"("State Variables in"=w467) -> ()  [unwired: 11 in]
    }
    frame #1 {
      n198 = invoke class="VI" method="FP.Close"() -> ()  [unwired: 3 in, 3 out]
    }
  }
